vi "Define Channel Count.vi"(8 "error in":errorcluster, 11 "NI 9474 in":refnum<class "NI 9474.lvclass">) -> (0 "error out":errorcluster, 3 "NI 9474 out":refnum<class "NI 9474.lvclass">)   [LabVIEW 2020, in "Scan Engine Scripting.lvlib" / "NI 9474.lvclass"]
uses:
  NI 9474.lvclass
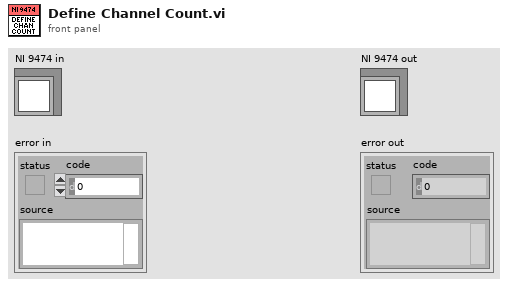
[diagram p1: front panel]
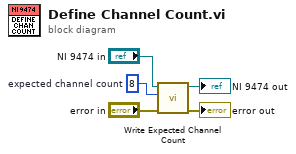
[diagram p0: block diagram]
diagram:
  w1 = 8  # expected channel count
  n1 = call-dynamic "Write Expected Channel Count.vi"("error in"="error in", "expected channel count"=w1, "module in"="NI 9474 in") -> ("error out"=→"error out":errorcluster, "module out"=→"NI 9474 out":refnum<class "NI 9474.lvclass">)  [unwired: 7 in]
